vi "Gen Help Tags.vi"(8 "error in (no error)":errorcluster, 11 "Context in":T1) -> (0 "error out":errorcluster, 3 "Context out":T1)   [LabVIEW 2020, in "DocTool.lvlib"]
uses:
  DocTool.lvlib
  TDefs/Context.ctl
  Events.ctl
  UserEvent.ctl
  TDefs/State.ctl
  TDefs/States.ctl
  TDefs/Single File Properties.ctl
  TDefs/FP Items Properties.ctl
  TDefs/FP Item Properties.ctl
  TDefs/CopyTag.ctl
  StateMachine.lvlib
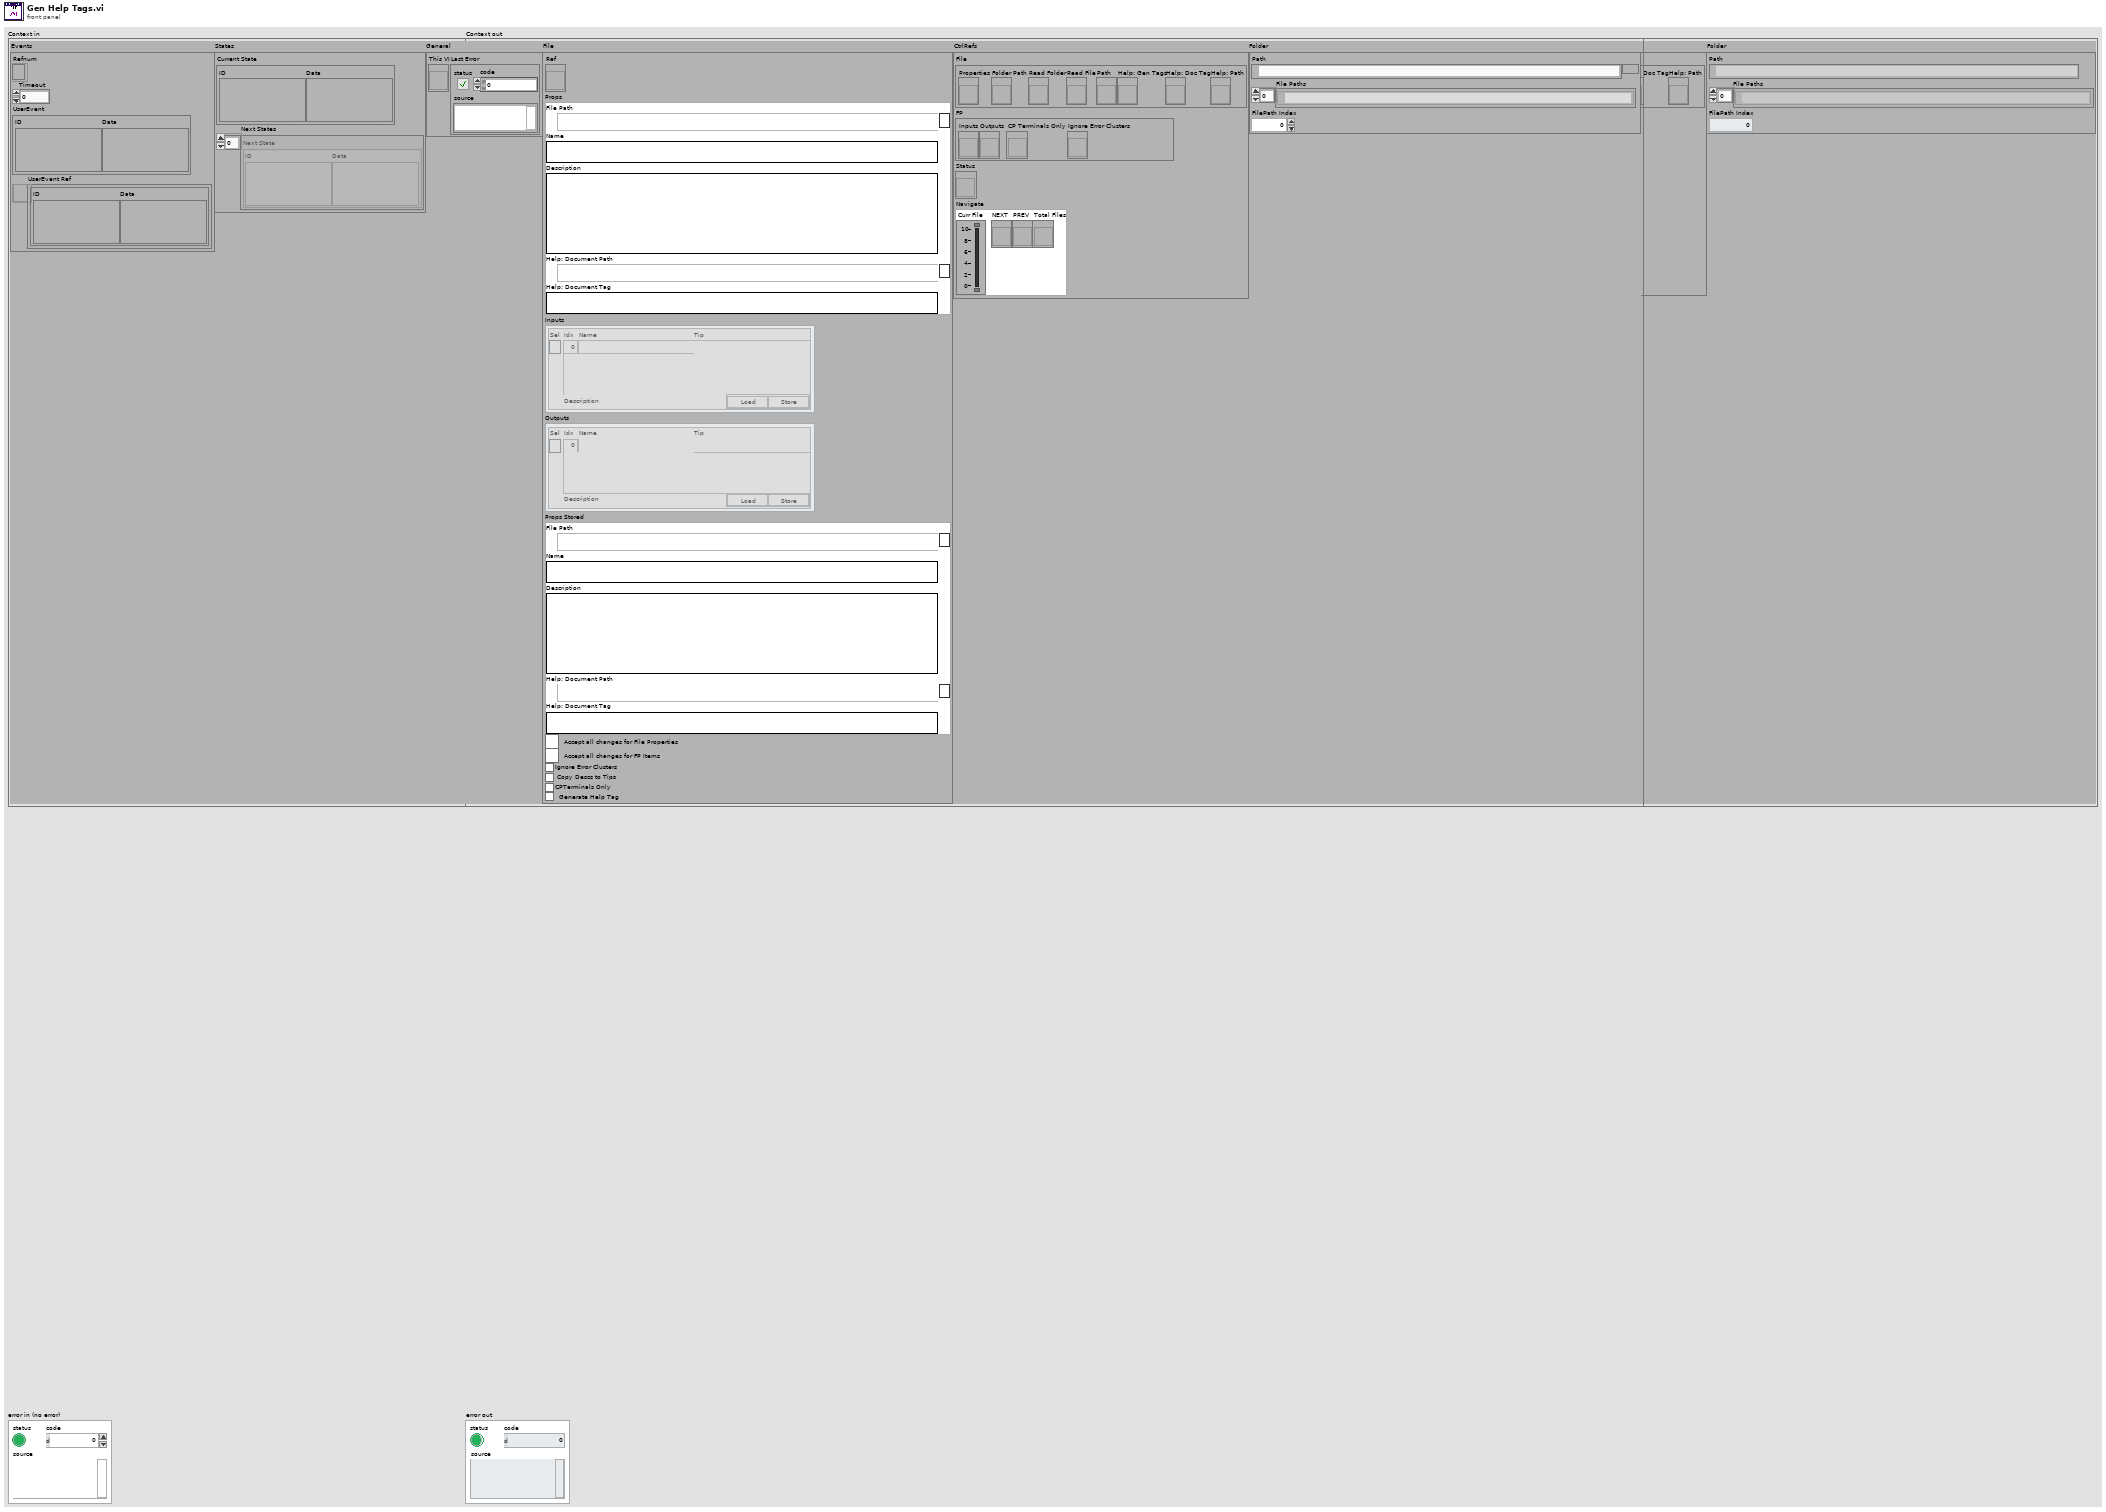
[diagram p1: front panel]
types:
  T1 = typedef "DocTool.lvlib/Context.ctl" = cluster{"Events":T2, "States":cluster{"Current State":T4, "Next States":T5}, "General":cluster{"This VI":refnum<vi>, "Last Error":errorcluster}, "File":cluster{"Ref":refnum<vi>, "Props":T6, "Inputs":T7, "Outputs":T7, "Props Stored":T6, "Write":bool, "Write FP":bool, "Ignore Error Clusters":bool, "Copy Descs to Tips":bool, "CPTerminals Only":bool, "Generate Help Tag":bool}, "CtrlRefs":cluster{"File":cluster{"Properties":refnum<vi>, "Folder Path":refnum<vi>, "Read Folder":refnum<vi>, "Read File":refnum<vi>, "Path":refnum<vi>, "Help: Gen Tags":refnum<vi>, "Help: Doc Tag":refnum<vi>, "Help: Path":refnum<vi>}, "FP":cluster{"Inputs":refnum<vi>, "Outputs":refnum<vi>, "CP Terminals Only":refnum<vi>, "Ignore Error Clusters":refnum<vi>}, "Status":refnum<vi>, "Navigate":cluster{"Curr File":refnum<vi>, "NEXT":refnum<vi>, "PREV":refnum<vi>, "Total Files":refnum<vi>}}, "Folder":cluster{"Path":path, "File Paths":path[], "FilePath Index":i32}}
  T2 = typedef "StateMachine.lvlib/Events.ctl" = cluster{"Refnum":refnum<event-registration>, "Timeout":i32, "UserEvent":T3, "UserEvent Ref":refnum<user-event>}
  T3 = typedef "StateMachine.lvlib/UserEvent.ctl" = cluster{"ID":variant, "Data":variant}
  T4 = typedef "StateMachine.lvlib/State.ctl" = cluster{"ID":variant, "Data":variant}
  T5 = typedef "StateMachine.lvlib/States.ctl" = T4[]
  T6 = typedef "DocTool.lvlib/Single File Properties.ctl" = cluster{"File Path":path, "Name":string, "Description":string, "Help: Document Path":path, "Help: Document Tag":string}
  T7 = typedef "DocTool.lvlib/FP Items Properties.ctl" = T8[]
  T8 = typedef "DocTool.lvlib/FP Item Properties.ctl" = cluster{"Sel":bool, "Idx":i32, "Name":string, "Description":string, "Tip":string, "Load Store":T9}
  T9 = typedef "DocTool.lvlib/CopyTag.ctl" = cluster{"Load":bool, "Store":bool}
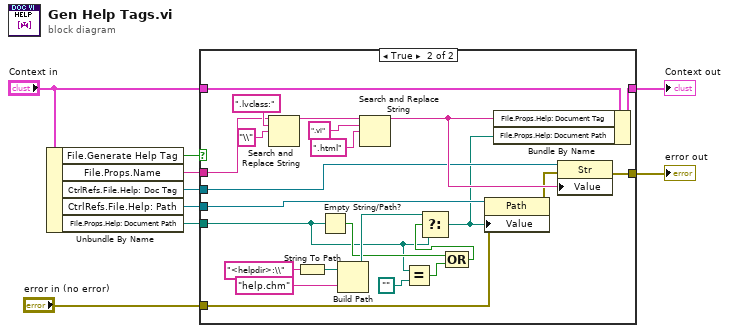
[diagram p0: block diagram]
diagram:
  n1 = Unbundle By Name("Context in") -> ("File.Generate Help Tag"=w9:bool, "File.Props.Name"=w1:string, "CtrlRefs.File.Help: Doc Tag"=w4:refnum<vi>, "CtrlRefs.File.Help: Path"=w6:refnum<vi>, "File.Props.Help: Document Path"=w5:path)
  n2 = case shown="True" w9 {
    tunnel: w1 -> [_ w30]
    tunnel: "Context in" -> [w11 w29]
    tunnel: [w11 w28] -> w3
    tunnel: w4 -> [_ w26]
    tunnel: w5 -> [_ w14]
    tunnel: w6 -> [_ w21]
    tunnel: "error in (no error)" -> [w10 w19]
    tunnel: [w10 w18] -> w8
    frame False {
    }
    frame True {
      n3 = Search and Replace String(input string=w30, search string=".lvclass:", replace string="\\" ("replace string (\"\")")) -> (result string=w33:string)  [unwired: 5 in, 3 out]
      n4 = String To Path(string="<helpdir>:\\") -> (path=w23:path)
      n5 = Empty String/Path?(string/path=w14) -> (empty?=w16:bool)
      n6 = Build Path(base path=w23, name or relative path="help.chm") -> (appended path=w22:path)
      n7 = Search and Replace String(input string=w33, search string=".vi", replace string=".html" ("search string")) -> (result string=w27:string)  [unwired: 5 in, 3 out]
      n8 = Equal?(x=w14, y=path "") -> (x = y?=w12:bool)
      n9 = Compound Arithmetic op=OR(w16, w12) -> (w15:bool)
      n10 = Select(t=w22, s=w15, f=w14) -> (s? t:f=w17:path)
      n11 = property on="Property Node" class="Path"(reference=w21, error in=w19, "Value"=w17) -> (error out=w20:errorcluster)  [unwired: 1 out]
      n12 = Bundle By Name(cluster=w29, "File.Props.Help: Document Tag"=w27, "File.Props.Help: Document Path"=w17) -> (w28:T1)
      n13 = property on="Property Node" class="Str"(reference=w26, error in=w20, "Value"=w27) -> (error out=w18:errorcluster)  [unwired: 1 out]
    }
  }
  "error out" <- w8
  "Context out" <- w3
